vi "Listbox-Set Checked Items.vi"(8 "error in (no error)":errorcluster, 9 "Checked Items":string[](array[string]), 11 "reference":refnum<vi>) -> (0 "error out":errorcluster)   [LabVIEW 2015]
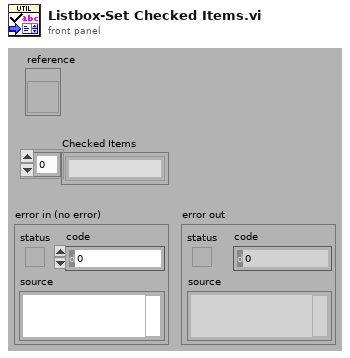
[diagram p1: front panel]
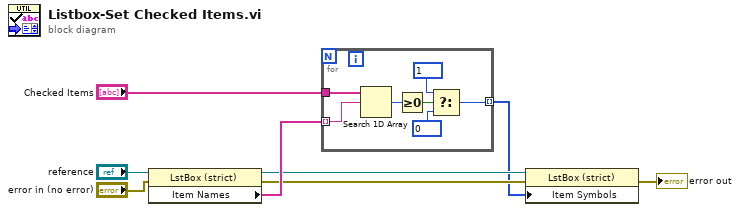
[diagram p0: block diagram]
diagram:
  n1 = property on="Property Node" class="LstBox (strict)"(reference="reference", error in="error in (no error)") -> (reference out=w4:refnum<vi>, error out=w3:errorcluster, "Item Names"=w8:string[])
  n2 = for {
    tunnel: w8 -> [w14] mode=indexing
    tunnel: "Checked Items" -> [w15]
    tunnel: [w9] -> w2 mode=indexing
    n3 = Search 1D Array(1D array=w15, element=w14) -> (index of element=w13:i32)  [unwired: 1 in]
    n4 = Greater Or Equal To 0?(x=w13) -> (x >= 0?=w12:bool)
    n5 = Select(t=1, s=w12, f=0) -> (s? t:f=w9:i32)
  }
  n6 = property on="Property Node" class="LstBox (strict)"(reference=w4, error in=w3, "Item Symbols"=w2) -> (error out=→"error out":errorcluster)  [unwired: 1 out]
